vi "Perform Action.vi"(8 "error in":errorcluster, 10 "Input":variant, 11 "AI DAQmx Cont CFG Simulated in":refnum<class "AI Current DAQmx Cont CFG Simulated.lvclass">) -> (0 "error out":errorcluster, 2 "Output":variant, 3 "AI DAQmx Cont CFG Simulated out":refnum<class "AI Current DAQmx Cont CFG Simulated.lvclass">)   [LabVIEW 2024, in "DAQmx Simulated CFGs.lvlib" / "AI Current DAQmx Cont CFG Simulated.lvclass"]
uses:
  AI Current DAQmx Cont CFG Simulated.lvclass
  DAQmx BufferLastReadsDBL/DAQmx BufferLastReadsDBL.lvclass/DAQmx BufferLastReadsDBL.ctl
  3231f087-4772-4f97-abee-d173a35e7553.vi
  <vilib>/JDP Science/JSONtext/Find Item.vi
  <vilib>/JDP Science/JSONtext/Next JSON Value.vi
  <vilib>/JDP Science/JSONtext/String Subset.vi
  <vilib>/JDP Science/JSONtext/Parsing/Advance past next JSON Value (inlined COPY).vi
  <vilib>/JDP Science/JSONtext/Parsing/Advance past whitespace.vi
  <vilib>/JDP Science/JSONtext/Parsing/Advance past String.vi
  <vilib>/JDP Science/JSONtext/Parsing/Advance past Number.vi
  <vilib>/JDP Science/JSONtext/Parsing/Advance past Line Ending.vi
  <vilib>/JDP Science/JSONtext/Parsing/Parse Full Path or Item Name.vi
  <vilib>/JDP Science/JSONtext/Parsing/Advance past Array.vi
  <vilib>/JDP Science/JSONtext/Parsing/Advance past Object.vi
  <vilib>/JDP Science/JSONtext/support/Error Cluster From Code.vi
  <vilib>/JDP Science/JSONtext/Offset/Find Item Locations by Path.vi
  <vilib>/JDP Science/JSONtext/JSON text to Variant.vi
  <vilib>/JDP Science/JSONtext/LVClass Serializer/JSONtext LVClass Serializer.lvclass
  DAQmx BufferLastReadsDBL/DAQmx BufferLastReadsDBL.lvclass
  Buffers/BufferLastReadingsDBL/BufferLastReadsDBL.lvclass
  Configurations/CFG JSON/CFG JSON.lvclass
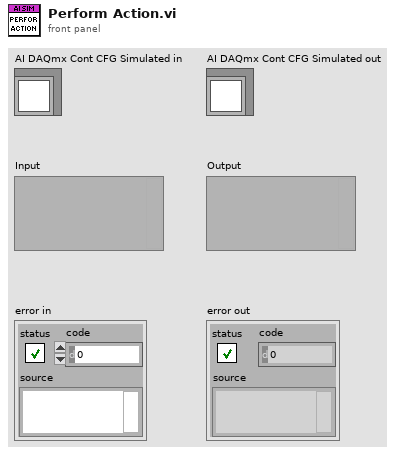
[diagram p1: front panel]
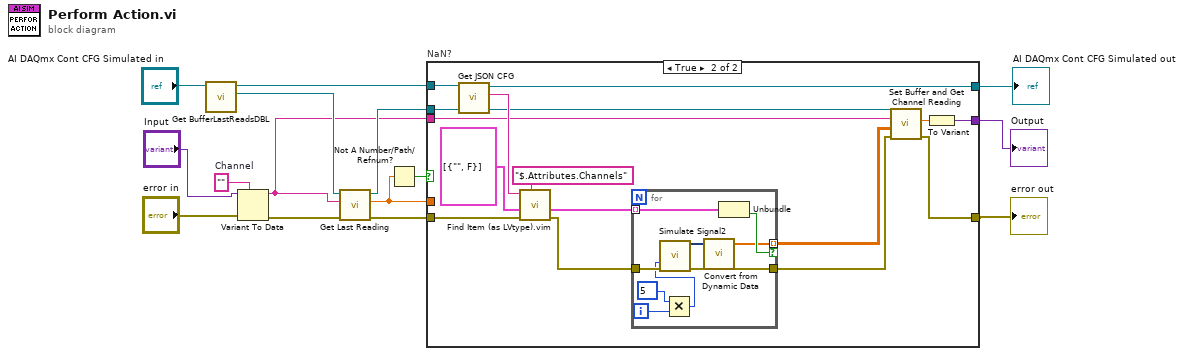
[diagram p0: block diagram]
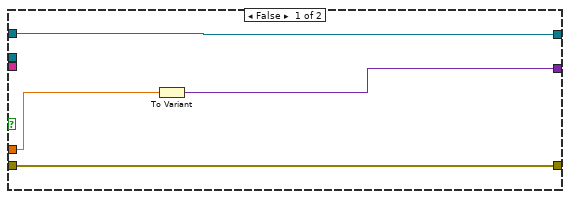
[diagram p2: hidden frame]
diagram:
  w3 = ""  # Channel
  n1 = call "Get BufferLastReadsDBL.vi"("DAQmx BufferLastReadsDBL in"="AI DAQmx Cont CFG Simulated in") -> ("BufferLastReadsDBL.lvclass"=w4:refnum<class "BufferLastReadsDBL.lvclass">, "DAQmx BufferLastReadsDBL out"=w5:refnum<class "AI Current DAQmx Cont CFG Simulated.lvclass">)  [unwired: 9 in]
  n2 = Variant To Data(error in="error in", type=w3, Variant="Input") -> (data=w2:string, error out=w1:errorcluster)
  n3 = call "Get Last Reading.vi"("error in"=w1, "Channel"=w2, "BufferLastReadingsDBL in"=w4) -> ("error out"=w14:errorcluster, "Reading"=w13:dbl, "BufferLastReadingsDBL out"=w11:refnum<class "BufferLastReadsDBL.lvclass">)  [unwired: 6 in]
  n4 = Not A Number/Path/Refnum?(number/path/refnum=w13) -> (NaN/Path/Refnum?=w15:bool)
  n5 = case "NaN?" shown="True" w15 {
    tunnel: w5 -> [w17 w34]
    tunnel: w14 -> [w16 w32]
    tunnel: [w16 w23] -> w7
    tunnel: [w18 w22] -> w10
    tunnel: [w17 w27] -> w8
    tunnel: w13 -> [w19 _]
    tunnel: w2 -> [_ w21]
    tunnel: w11 -> [_ w26]
    frame False {
      n6 = To Variant(anything=w19) -> (Variant=w18:variant)
    }
    frame True {
      n7 = call "Get JSON CFG.vi"("CFG JSON in"=w34) -> ("<JSON> CFG"=w33:string, "CFG JSON out"=w27:refnum<class "AI Current DAQmx Cont CFG Simulated.lvclass">)  [unwired: 9 in]
      n8 = call "Find Item (as LVtype).vim"("$Path or Item Name"="$.Attributes.Channels", "error in (no error)"=w32, "Data Type and Default Value"=cluster{"Name":string, "Enabled":bool}[] [{"Name"="", "Enabled"=FALSE}], "JSON"=w33) -> ("error out"=w28:errorcluster, "Data"=w29:cluster{"Name":string, "Enabled":bool}[])  [unwired: 4 in, 2 out]
      n9 = for {
        tunnel: w29 -> [w43] mode=indexing
        tunnel: w28 -> [w42]
        tunnel: [w41] -> w24
        tunnel: [w36] -> w25 mode=indexing if=w40
        i -> [w39]
        n10 = Multiply(x=5, y=w39) -> (x*y=w35:i32)
        n11 = call "Simulate Signal2"("Phase"=w35, "error in (no error)"=w42) -> ("Sine with Uniform Noise"=w37:dynamicdata, "error out"=w41:errorcluster)  [unwired: 12 in]
        n12 = call "Convert from Dynamic Data"("Dynamic Data Type"=w37) -> ("Array"=w36:dbl[])  [unwired: 3 in]
        n13 = Unbundle(w43) -> ("Enabled"=w40:bool)  [unwired: 1 out]
      }
      n14 = call "Set Buffer and Get Channel Reading.vi"("error in"=w24, "Readings"=w25, "Channel Ident"=w21, "BufferLastReadingsDBL in"=w26) -> ("error out"=w23:errorcluster, "Reading"=w20:dbl)  [unwired: 5 in, 1 out]
      n15 = To Variant(anything=w20) -> (Variant=w22:variant)
    }
  }
  "error out" <- w7
  "AI DAQmx Cont CFG Simulated out" <- w8
  "Output" <- w10
